vi "Main.vi"() -> ()   [LabVIEW 2017]
doc: "Use this template to build a simple state machine design pattern. Each state executes code and determines which state to transition to."
uses:
  Controls/State.ctl
  Controls/Data.ctl
  Controls/Database_Array.ctl
  Controls/Encoding.ctl
  <vilib>/Utility/error.llb/DialogType.ctl
  <userlib>/_OpenG.lib/array/array.llb/Remove Duplicates from 1D Array (I32)__ogtk.vi
  <userlib>/_OpenG.lib/array/array.llb/Sort 1D Array (I32)__ogtk.vi
  <userlib>/_OpenG.lib/array/array.llb/Search 1D Array (I32)__ogtk.vi
  <userlib>/_OpenG.lib/array/array.llb/Index 1D Array Elements (Variant)__ogtk.vi
panel:
  out "Progress":string
  in  "Stop Button":bool
  in  "Generate XMLs":bool
  in  "Database Filepath (xlsx)":path
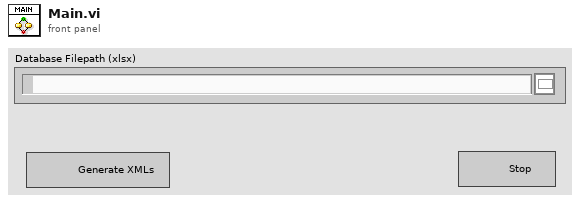
[diagram p1: front panel]
types:
  T1 = typedef "DialogType.ctl" = u16
  T2 = typedef "Data.ctl" = cluster{"Cores to Process Array":i32[], "All Parameters Array":T3[], "Filtered Parameter Array":T3[], "Core Number":i32, "Database Filepath (xlsx)":path}
  T3 = typedef "Database_Array.ctl" = cluster{"Core Number":i32, "Channel Number":i32, "Channel Name":string, "Channel Speed":i32, "Label Decimal":i32, "Label Name":string, "Min Rate (mS)":i32, "Max Rate (mS)":i32, "SDI":i32, "SSM":i32, "Create SDI":bool, "Create SSM":bool, "Create Parity":bool, "Parameter Name":string, "Start Bit":i32, "Number of Bits":i32, "Scale":string, "Offset":string, "Signed":bool, "Unit":string, "Encoding":T4, "Default Value":string}
  T4 = typedef "Encoding.ctl" = enum16{"BCD", "BNR", "Discrete"}
  T5 = typedef "State.ctl" = enum16{"Initialize", "Wait for Event", "Read Database File", "Get Core Data", "Write HW XML File", "Write Parameter XML File", "HW XML - Close", "User State 2", "Exit"}
  T6 = enum8{"Enabled", "Disabled", "Disabled and Grayed Out"}
  T7 = enum32{"invalid app kind", "Development System", "Run Time System", "Student Edition", "Embedded LabVIEW", "Evaluation", "Custom"}
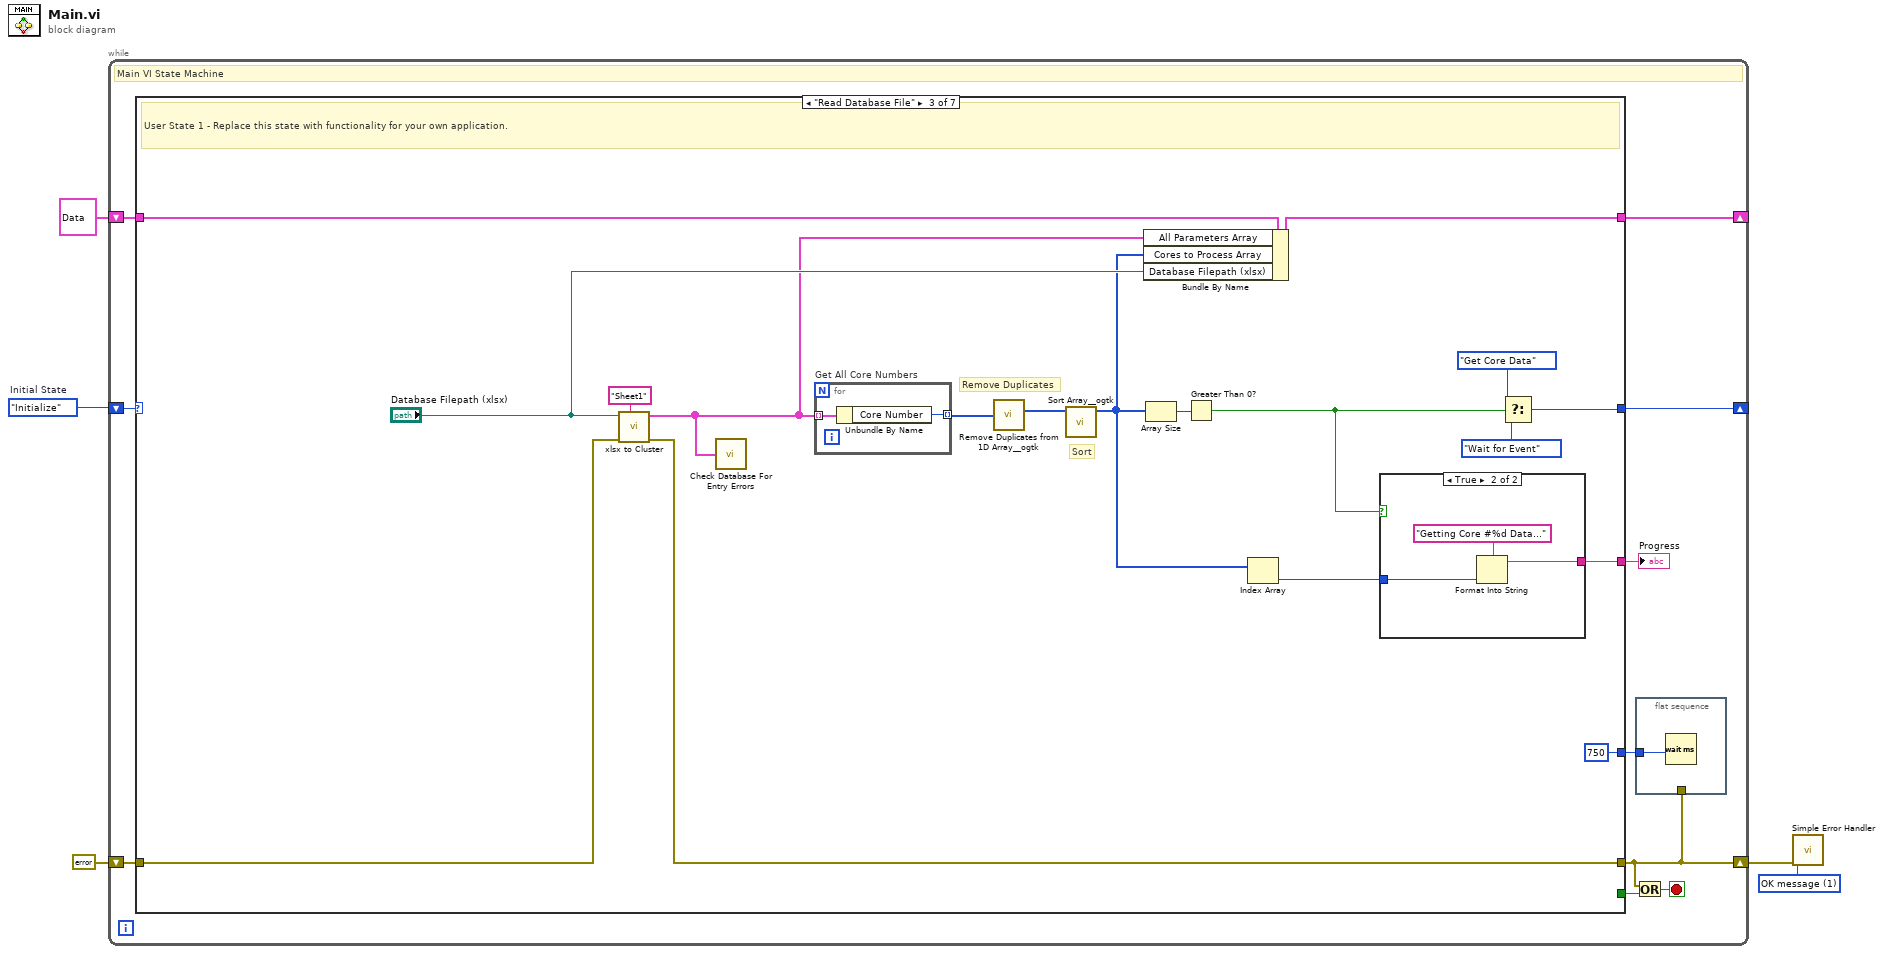
[diagram p0: block diagram]
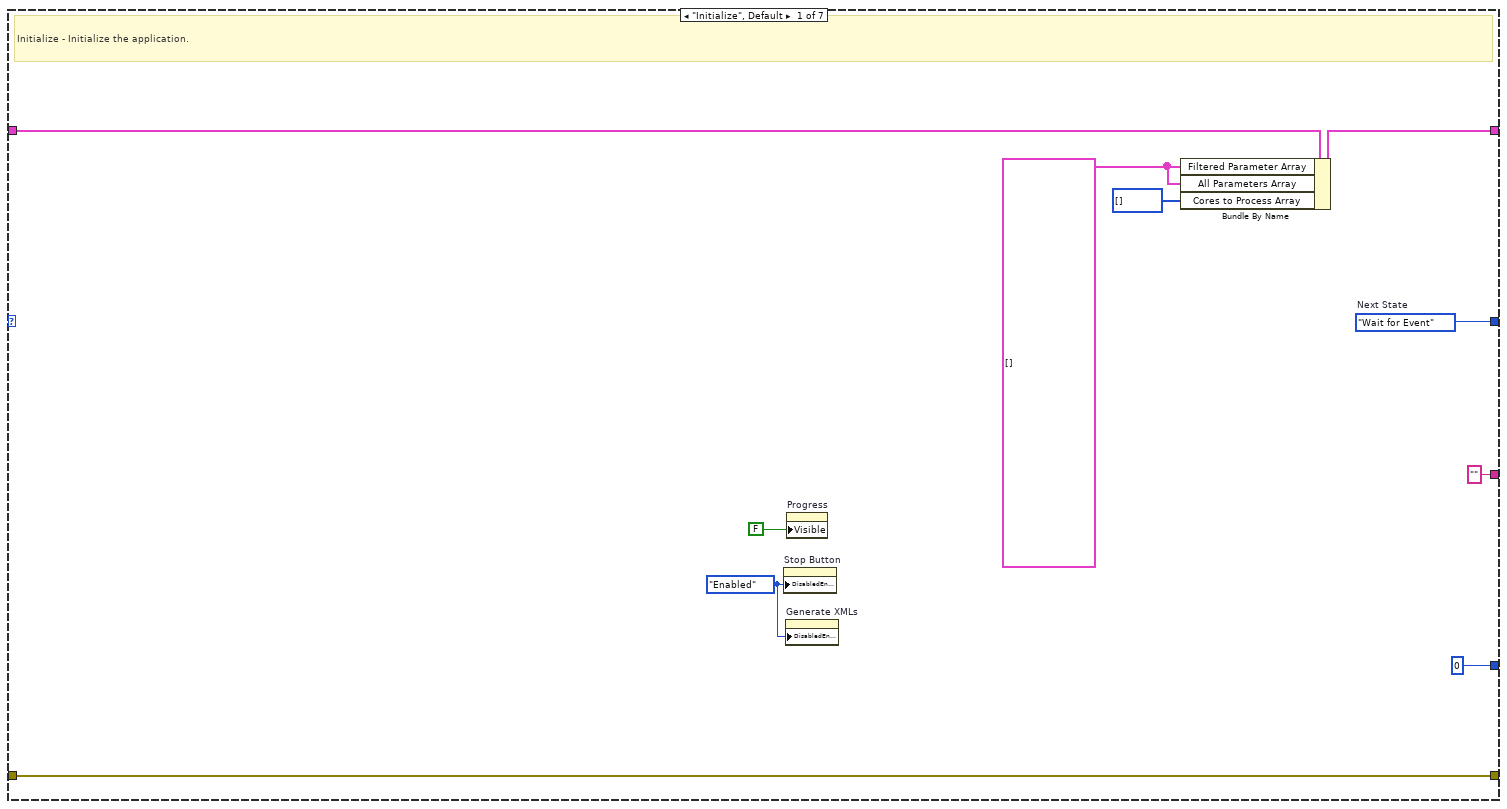
[diagram p2: hidden frame]
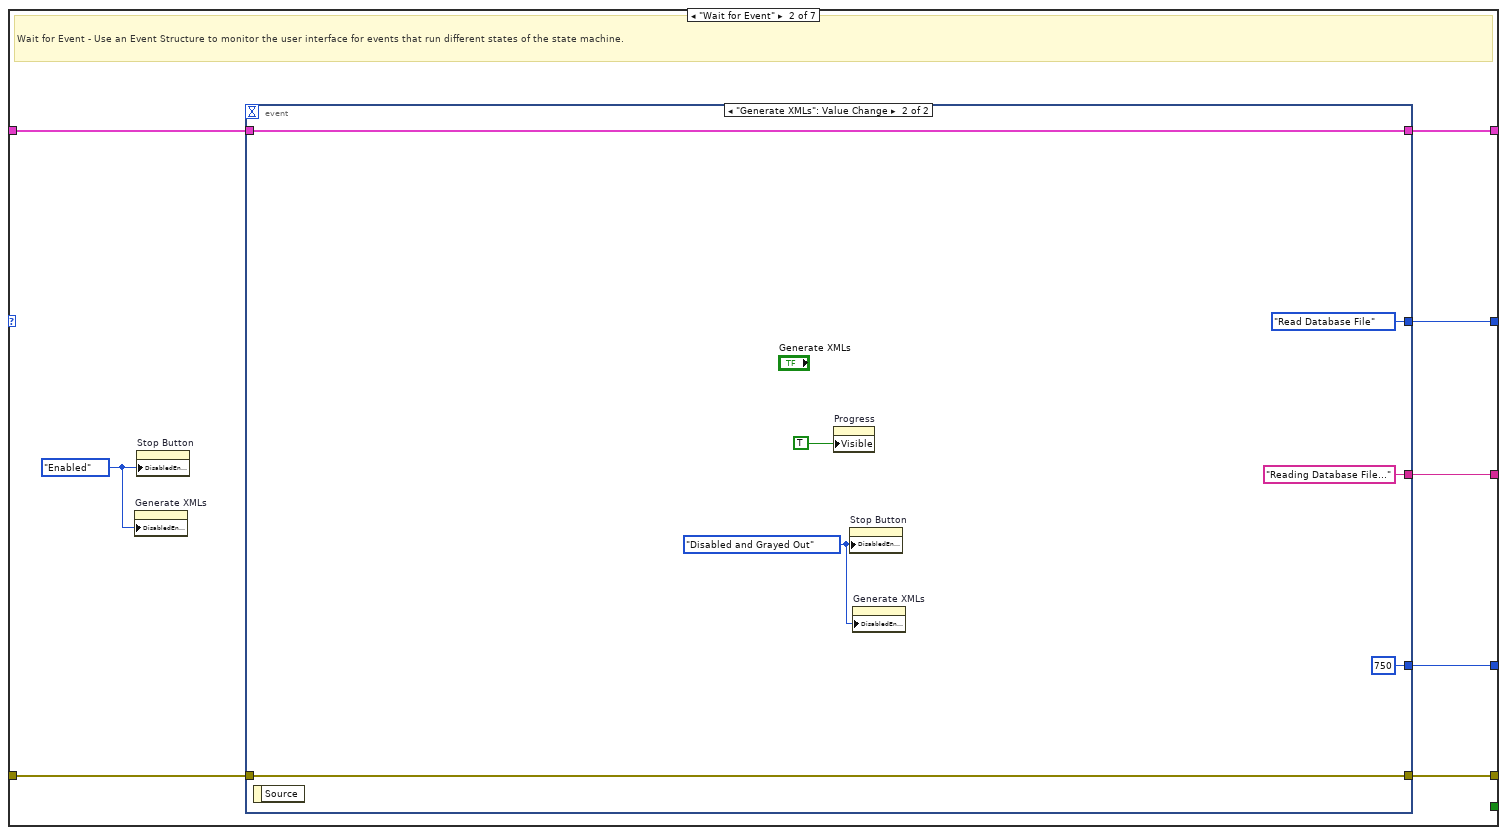
[diagram p3: hidden frame]
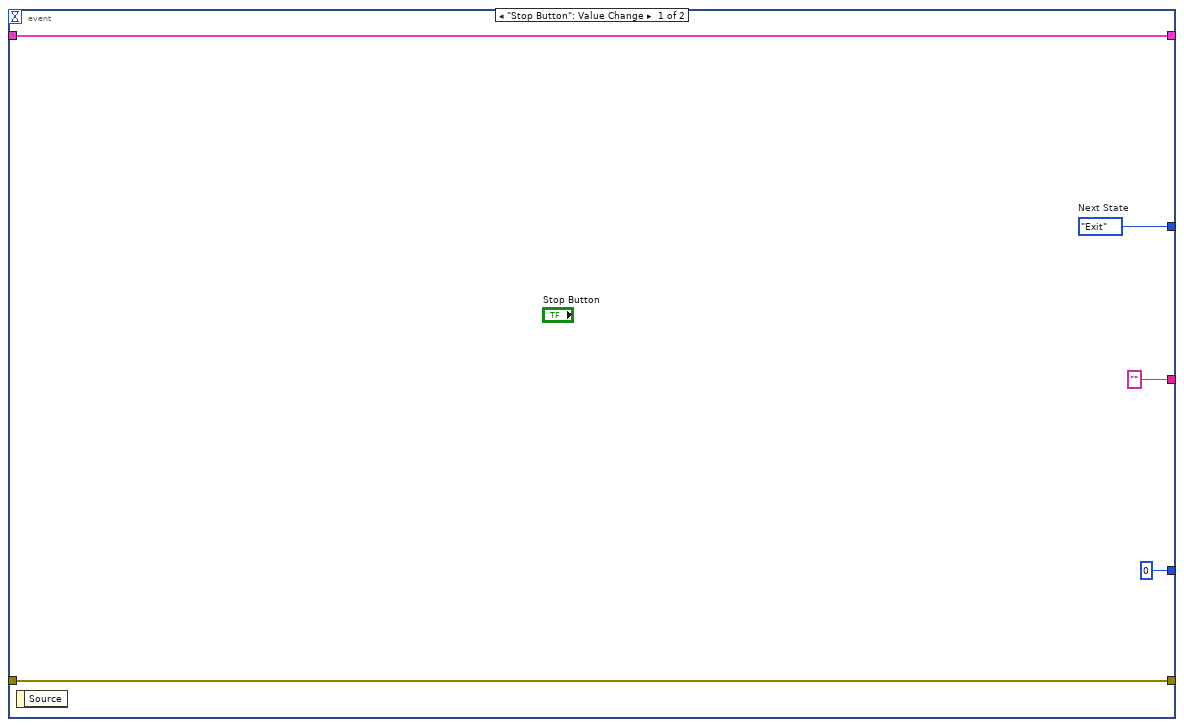
[diagram p4: hidden frame]
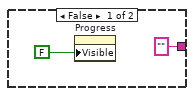
[diagram p5: hidden frame]
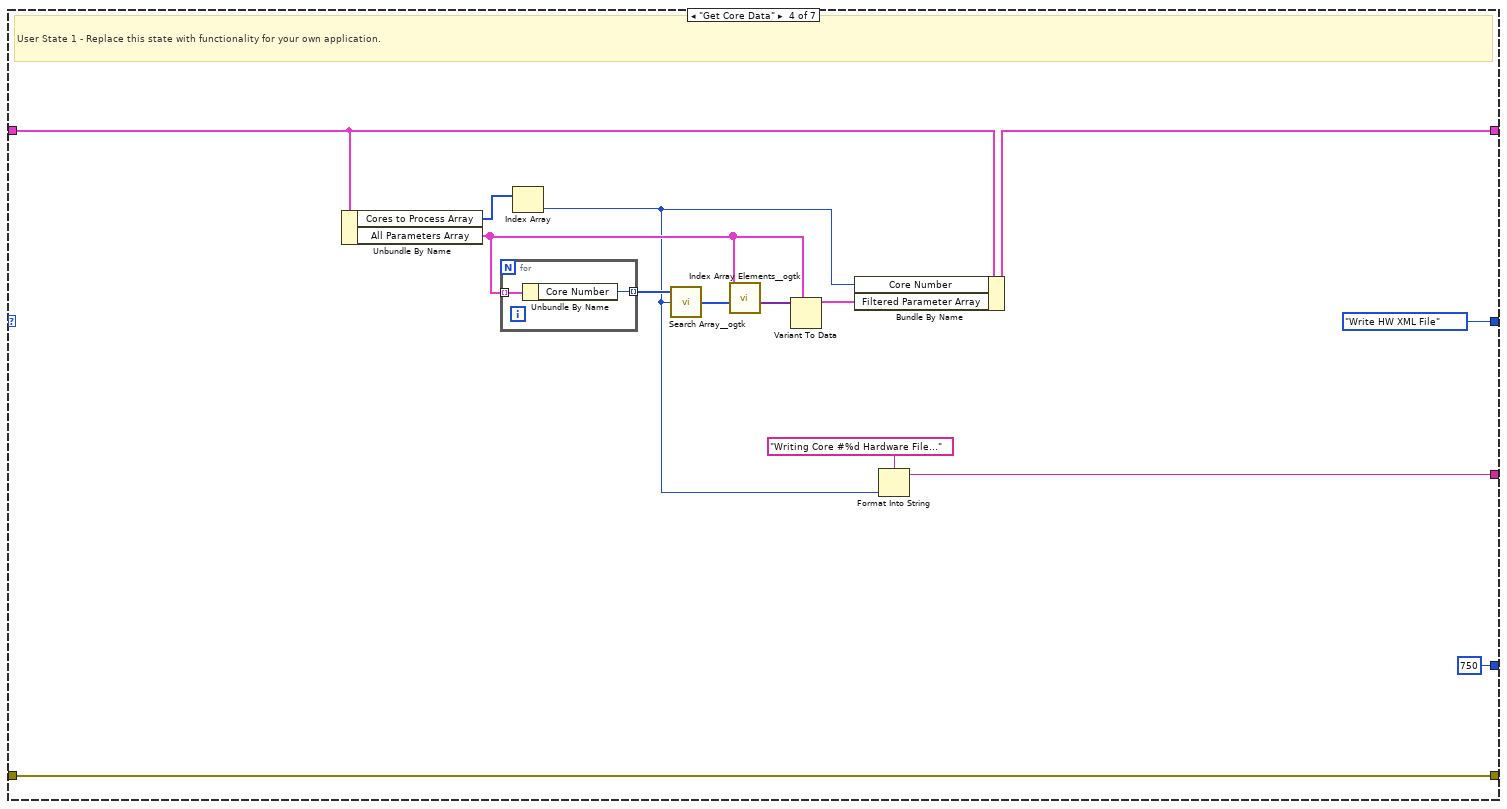
[diagram p6: hidden frame]
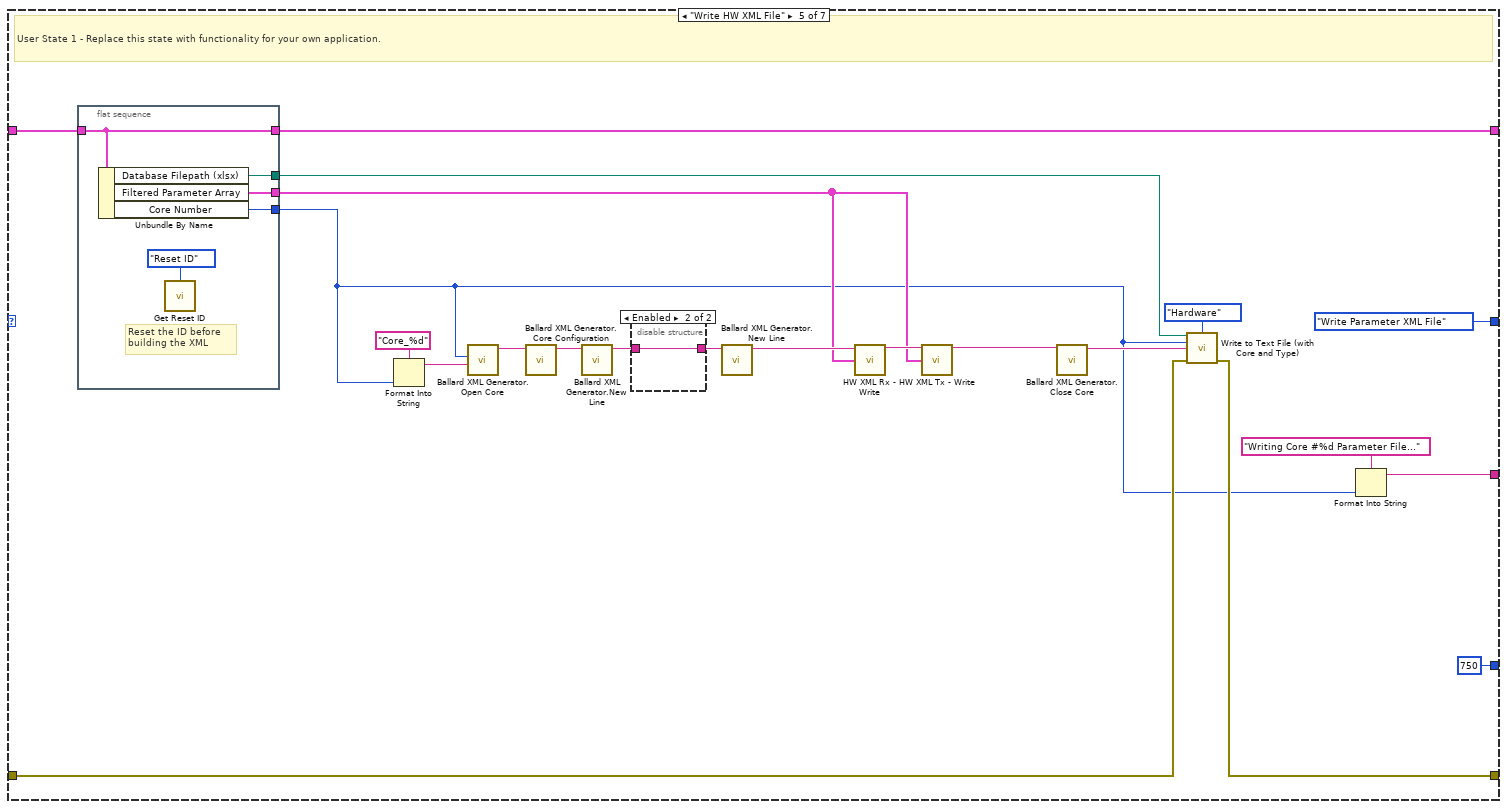
[diagram p7: hidden frame]
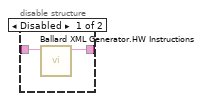
[diagram p8: hidden frame]
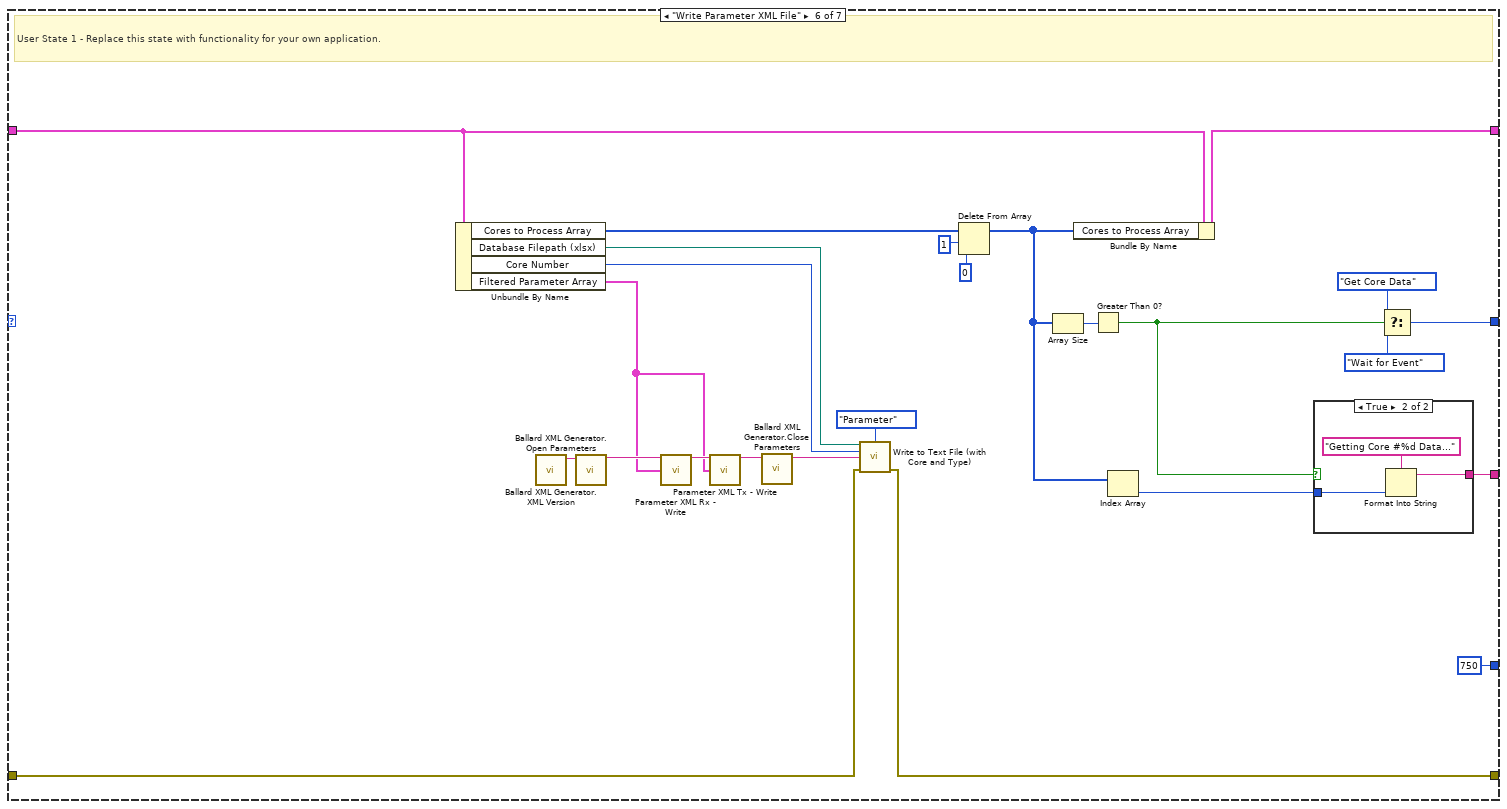
[diagram p9: hidden frame]
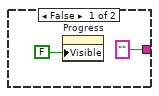
[diagram p10: hidden frame]
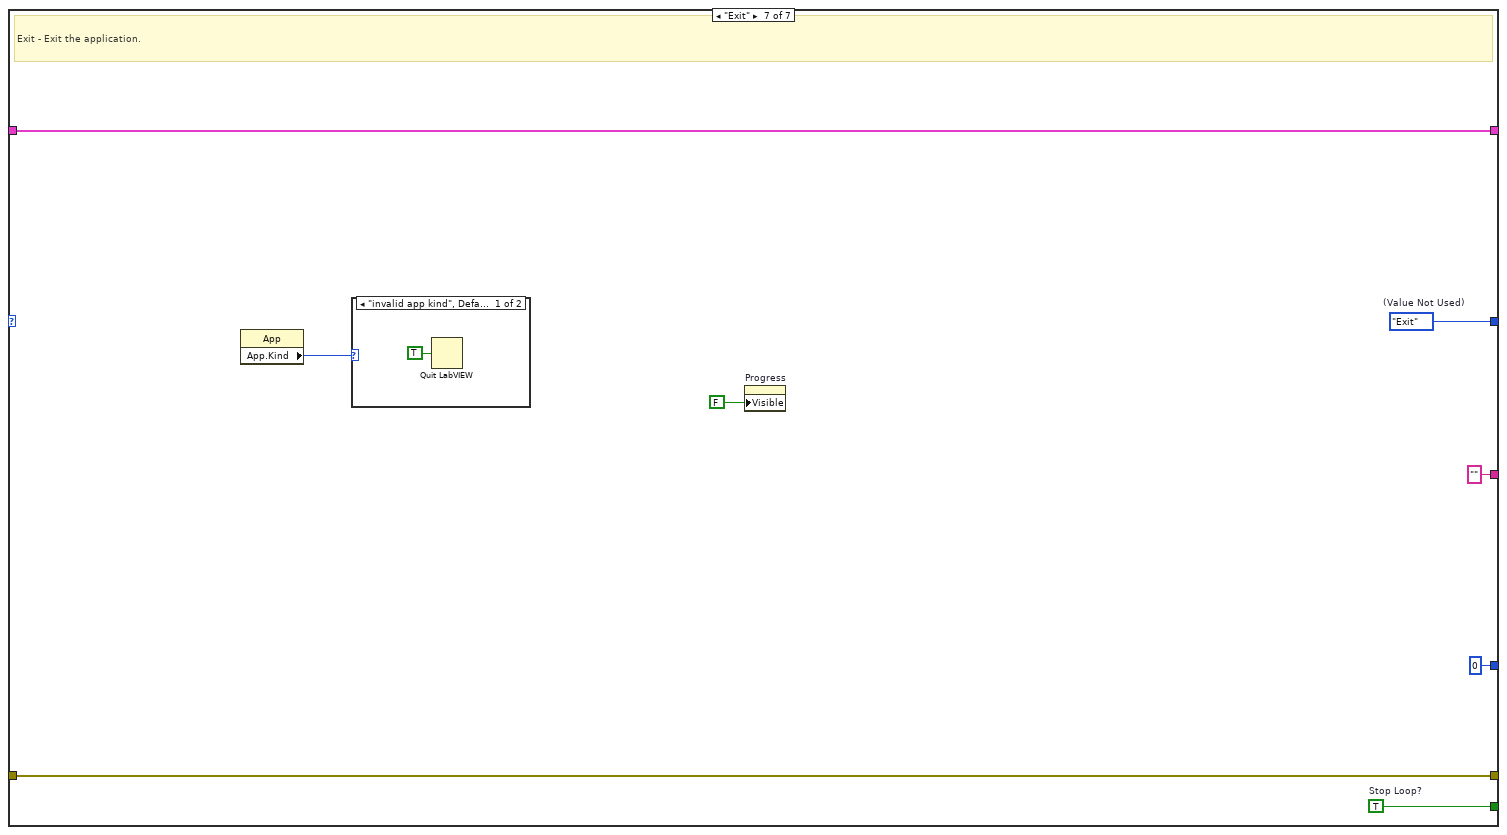
[diagram p11: hidden frame]
diagram:
  w1 = T1 1 items=["no dialog", "OK message", "continue or stop message", "OK message + warnings", "continue/stop + warnings"] ("type of dialog (OK msg:1)")
  w5 = State."Initialize"  # Initial State
  n1 = while {
    shift-right: [w14] -> _
    shift-left: w5 -> [w15]
    shift-right: [w12] -> _
    shift-left: T2 {"Cores to Process Array"=[], "All Parameters Array"=[], "Filtered Parameter Array"=[], "Core Number"=0, "Database Filepath (xlsx)"=path "C:/Users/jkreienh/Desktop/Preliminary Ballard Database Template.xlsx"} ("Data") -> [w13]
    shift-right: [w7] -> w2
    shift-left: errorcluster {"status"=FALSE, "code"=0, "source"=""} ("error constant") -> [w11]
    stop <- w9 stop-if-true
    # "Main VI State Machine"
    n2 = case shown="\"Read Database File\"" w15 {
      tunnel: [w26 w34 w55 State."Write HW XML File" State."Write Parameter XML File" ("Next State") w133 w155] -> w14
      tunnel: [_ _ _ _ _ _ w153] -> w10
      tunnel: w13 -> [w24 w33 w60 w82 w94 w130 w154]
      tunnel: [w23 w32 w59 w85 w93 w129 w154] -> w12
      tunnel: w11 -> [w25 w31 w52 w76 w97 w138 w152]
      tunnel: [w25 w30 w63 w76 w96 w137 w152] -> w7
      tunnel: ["" w29 w51 w73 w89 w123 ""] -> w8
      tunnel: [u32 0 ("milliseconds to wait") w28 u32 750 ("milliseconds to wait") u32 750 ("milliseconds to wait") u32 750 ("milliseconds to wait") u32 750 ("milliseconds to wait") u32 0 ("milliseconds to wait")] -> w6
      frame "Initialize", Default {
        w17 = T6."Enabled" ("Disabled")
        w21 = T3[] [] ("Parameter Array")
        w26 = State."Wait for Event"  # Next State
        # "Initialize - Initialize the application."
        n3 = property on="Stop Button" class="Bool"("DisabledEnum"=w17) -> ()  [unwired: 2 in, 2 out]
        n4 = property on="Generate XMLs" class="Bool"("DisabledEnum"=w17) -> ()  [unwired: 2 in, 2 out]
        n5 = property on="Progress" class="Str"("Visible"=FALSE) -> ()  [unwired: 2 in, 2 out]
        n6 = Bundle By Name(cluster=w24, "Filtered Parameter Array"=w21, "All Parameters Array"=w21, "Cores to Process Array"=i32[] [] ("Core Array")) -> (w23:T2)
      }
      frame "Wait for Event" {
        w27 = T6."Enabled" ("Disabled")
        # "Wait for Event - Use an Event Structure to monitor the user interface for events that run different states of the state machine."
        n7 = property on="Generate XMLs" class="Bool"("DisabledEnum"=w27) -> ()  [unwired: 2 in, 2 out]
        n8 = property on="Stop Button" class="Bool"("DisabledEnum"=w27) -> ()  [unwired: 2 in, 2 out]
        n9 = event shown="[1] \"Generate XMLs\": Value Change" {
          selector: _ -> [_ _]
          dyn-events: _ -> [_ _]
          timeout: _ -> [_ _]
          tunnel: [w39 State."Read Database File" ("Next State")] -> w34
          tunnel: w33 -> [w38 w46]
          tunnel: [w38 w46] -> w32
          tunnel: w31 -> [w37 w45]
          tunnel: [w37 w45] -> w30
          tunnel: ["" "Reading Database File..."] -> w29
          tunnel: [u32 0 ("milliseconds to wait") u32 750 ("milliseconds to wait")] -> w28
          event "Stop Button": Value Change {
            w39 = State."Exit"  # Next State
            n10 = event-data() -> ()  [unwired: 1 in, 1 out]
          }
          event "Generate XMLs": Value Change {
            w40 = T6."Disabled and Grayed Out" ("Disabled")
            n11 = event-data() -> ()  [unwired: 1 in, 1 out]
            n12 = property on="Progress" class="Str"("Visible"=TRUE) -> ()  [unwired: 2 in, 2 out]
            n13 = property on="Stop Button" class="Bool"("DisabledEnum"=w40) -> ()  [unwired: 2 in, 2 out]
            n14 = property on="Generate XMLs" class="Bool"("DisabledEnum"=w40) -> ()  [unwired: 2 in, 2 out]
          }
        }
      }
      frame "Read Database File" {
        # "Sort"
        # "Remove Duplicates"
        # "User State 1 - Replace this state with functionality for your own application."
        n15 = call "xlsx to Cluster.vi"("Excel._SheetName"="Sheet1", "Error (in)"=w52, "file path (dialog if empty)"="Database Filepath (xlsx)") -> ("Error (out)"=w63:errorcluster, "Parameter Array"=w53:T3[])  [unwired: 7 in]
        n16 = call "Check Database For Entry Errors.vi"("All Parameters Array"=w53) -> ()  [unwired: 15 in]
        n17 = for "Get All Core Numbers" {
          tunnel: w53 -> [w71] mode=indexing
          tunnel: [w70] -> w62 mode=indexing
          n18 = Unbundle By Name(w71) -> ("Core Number"=w70:i32)
        }
        n19 = call-poly <userlib>:"Remove Duplicates from 1D Array__ogtk.vi"("Input Array"=w62) -> ("Output Array"=w61:i32[])  [unwired: 1 out]
        n20 = call-poly <userlib>:"Sort Array__ogtk.vi"("Array in"=w61) -> ("Sorted Array out"=w50:i32[])  [unwired: 9 in, 1 out]
        n21 = Bundle By Name(cluster=w60, "All Parameters Array"=w53, "Cores to Process Array"=w50, "Database Filepath (xlsx)"="Database Filepath (xlsx)") -> (w59:T2)
        n22 = Array Size(array=w50) -> (size(s)=w58:i32)
        n23 = Greater Than 0?(x=w58) -> (x > 0?=w48:bool)
        n24 = Index Array(array=w50) -> (element=w49:i32)  [unwired: 1 in]
        n25 = case shown="True" w48 {
          tunnel: ["" ("f") w68] -> w51
          tunnel: w49 -> [_ w69]
          frame False {
            n26 = property on="Progress" class="Str"("Visible"=FALSE) -> ()  [unwired: 2 in, 2 out]
          }
          frame True {
            n27 = Format Into String(format string="Getting Core #%d Data..." ("String"), w69) -> (resulting string=w68:string)  [unwired: 2 in, 1 out]
          }
        }
        n28 = Select(t=State."Get Core Data", s=w48, f=State."Wait for Event") -> (s? t:f=w55:T5)
      }
      frame "Get Core Data" {
        # "User State 1 - Replace this state with functionality for your own application."
        n29 = Unbundle By Name(w82) -> ("Cores to Process Array"=w78:i32[], "All Parameters Array"=w81:T3[])
        n30 = for {
          tunnel: w81 -> [w87] mode=indexing
          tunnel: [w86] -> w84 mode=indexing
          n31 = Unbundle By Name(w87) -> ("Core Number"=w86:i32)
        }
        n32 = Index Array(array=w78) -> (element=w74:i32)  [unwired: 1 in]
        n33 = call-poly <userlib>:"Search Array__ogtk.vi"("Array"=w84, "Element Data"=w74) -> ("Indices of Elements"=w83:i32[])  [unwired: 7 in]
        n34 = call-poly <userlib>:"Index Array Elements__ogtk.vi"("indices"=w83, "array"=w81) -> ("elements"=w80:variant[])  [unwired: 9 in]
        n35 = Variant To Data(type=w81, Variant=w80) -> (data=w79:T3[])  [unwired: 1 in, 1 out]
        n36 = Bundle By Name(cluster=w82, "Core Number"=w74, "Filtered Parameter Array"=w79) -> (w85:T2)
        n37 = Format Into String(format string="Writing Core #%d Hardware File..." ("String"), w74) -> (resulting string=w73:string)  [unwired: 2 in, 1 out]
      }
      frame "Write HW XML File" {
        # "User State 1 - Replace this state with functionality for your own application."
        n38 = flat-sequence {
          tunnel: [w114] -> w99
          tunnel: w94 -> [w111]
          tunnel: [w113] -> w90
          tunnel: [w111] -> w93
          tunnel: [w110] -> w92
          frame #0 {
            # "Reset the ID before building the XML"
            n39 = Unbundle By Name(w111) -> ("Database Filepath (xlsx)"=w110:path, "Filtered Parameter Array"=w114:T3[], "Core Number"=w113:i32)
            n40 = call "Get Reset ID.vi"("Function"=enum16{"Get ID", "Reset ID"}."Reset ID") -> ()  [unwired: 14 in, 1 out]
          }
        }
        n41 = Format Into String(format string="Core_%d", w90) -> (resulting string=w100:string)  [unwired: 2 in, 1 out]
        n42 = call "Ballard XML Generator.Open Core.vi"("name"=w100, "id"=w90) -> ("string out"=w102:string)  [unwired: 9 in]
        n43 = call "Ballard XML Generator.Core Configuration.vi"("string in"=w102) -> ("string out"=w103:string)  [unwired: 10 in]
        n44 = call "Ballard XML Generator.New Line.vi"("string in"=w103) -> ("string out"=w104:string)  [unwired: 10 in]
        n45 = disable-structure shown="Enabled" {
          disable-tunnel: w104 -> [w116 w117]
          disable-tunnel: [w115 w117] -> w105
          frame Disabled {
            n46 = call "Ballard XML Generator.HW Instructions.vi"("string in"=w116) -> ("string out"=w115:string)  [unwired: 10 in]
          }
          frame Enabled {
          }
        }
        n47 = call "Ballard XML Generator.New Line.vi"("string in"=w105) -> ("string out"=w106:string)  [unwired: 10 in]
        n48 = call "HW XML Rx - Write.vi"("String (in)"=w106, "Parameter Array"=w99) -> ("String (out)"=w107:string)  [unwired: 13 in]
        n49 = call "HW XML Tx - Write.vi"("String (in)"=w107, "Parameter Array"=w99) -> ("String (out)"=w108:string)  [unwired: 13 in]
        n50 = call "Ballard XML Generator.Close Core.vi"("string in"=w108) -> ("string out"=w95:string)  [unwired: 10 in]
        n51 = call "Write to Text File (with Core and Type).vi"("Database Filepath (xlsx)"=w92, "Filetype"=enum16{"Hardware", "Parameter"}."Hardware", "Core"=w90, "Text"=w95, "Error (in)"=w97) -> ("Error (out)"=w96:errorcluster)  [unwired: 10 in]
        n52 = Format Into String(format string="Writing Core #%d Parameter File..." ("String"), w90) -> (resulting string=w89:string)  [unwired: 2 in, 1 out]
      }
      frame "Write Parameter XML File" {
        # "User State 1 - Replace this state with functionality for your own application."
        n53 = Unbundle By Name(w130) -> ("Cores to Process Array"=w131:i32[], "Database Filepath (xlsx)"=w125:path, "Core Number"=w122:i32, "Filtered Parameter Array"=w126:T3[])
        n54 = call "Ballard XML Generator.XML Version.vi"() -> ("string out"=w142:string)  [unwired: 11 in]
        n55 = call "Ballard XML Generator.Open Parameters.vi"("string in"=w142) -> ("string out"=w141:string)  [unwired: 10 in]
        n56 = call "Parameter XML Rx - Write.vi"("String (in)"=w141, "Parameter Array"=w126) -> ("String (out)"=w140:string)  [unwired: 13 in]
        n57 = call "Parameter XML Tx - Write.vi"("String (in)"=w140, "Parameter Array"=w126) -> ("String (out)"=w139:string)  [unwired: 13 in]
        n58 = call "Ballard XML Generator.Close Parameters.vi"("string in"=w139) -> ("string out"=w128:string)  [unwired: 10 in]
        n59 = call "Write to Text File (with Core and Type).vi"("Database Filepath (xlsx)"=w125, "Filetype"=enum16{"Hardware", "Parameter"}."Parameter", "Core"=w122, "Text"=w128, "Error (in)"=w138) -> ("Error (out)"=w137:errorcluster)  [unwired: 10 in]
        n60 = Delete From Array(array=w131, length=1, index=0) -> (array with subset deleted=w120:i32[])  [unwired: 1 out]
        n61 = Array Size(array=w120) -> (size(s)=w136:i32)
        n62 = Bundle By Name(cluster=w130, "Cores to Process Array"=w120) -> (w129:T2)
        n63 = Greater Than 0?(x=w136) -> (x > 0?=w121:bool)
        n64 = Index Array(array=w120) -> (element=w119:i32)  [unwired: 1 in]
        n65 = case shown="True" w121 {
          tunnel: ["" w146] -> w123
          tunnel: w119 -> [_ w145]
          frame False {
            n66 = property on="Progress" class="Str"("Visible"=FALSE) -> ()  [unwired: 2 in, 2 out]
          }
          frame True {
            n67 = Format Into String(format string="Getting Core #%d Data..." ("String"), w145) -> (resulting string=w146:string)  [unwired: 2 in, 1 out]
          }
        }
        n68 = Select(t=State."Get Core Data" ("Next State"), s=w121, f=State."Wait for Event" ("Next State")) -> (s? t:f=w133:T5)
      }
      frame "Exit" {
        w153 = TRUE  # Stop Loop?
        w155 = State."Exit"  # (Value Not Used)
        # "Exit - Exit the application."
        n69 = property class="App"() -> ("App.Kind"=w148:T7)  [unwired: 2 in, 2 out]
        n70 = case shown="\"invalid app kind\", Default" w148 {
          frame "invalid app kind", Default {
            n71 = Quit LabVIEW(quit? (T)=TRUE) -> ()
          }
          frame "Development System" {
          }
        }
        n72 = property on="Progress" class="Str"("Visible"=FALSE) -> ()  [unwired: 2 in, 2 out]
      }
    }
    "Progress" <- w8
    n73 = Or(x=w7, y=w10) -> (x .or. y?=w9:bool)
    n74 = flat-sequence {
      tunnel: w7 -> [_]
      tunnel: w6 -> [w16]
      frame #0 {
        n75 = Wait (ms)(milliseconds to wait=w16) -> ()  [unwired: 1 out]
      }
    }
  }
  n76 = call <vilib>:"Simple Error Handler.vi"("type of dialog (OK msg:1)"=w1, "error in (no error)"=w2) -> ()  [unwired: 3 in, 5 out]
